vi "Configure QQ.vi"(8 "error in (no error)":errorcluster, 9 "Q / Q High (5 V)":dbl=5.0, 10 "Q / Q Low (0 V)":dbl, 11 "VISA resource name":refnum<visa-resource-name>) -> (0 "error out":errorcluster, 3 "VISA resource name out":refnum<visa-resource-name>)   [LabVIEW 2013, in "Stanford Research CG635.lvlib"]
doc: "Set the Q / Q <b>high</b> and <b>low</b> controls to the specified values.\n\n<b>Note</b>: for standard values/levels, use the Configure Standard Outputs VI."
uses:
  <instrlib>/Stanford Research CG635/Stanford Research CG635.lvlib
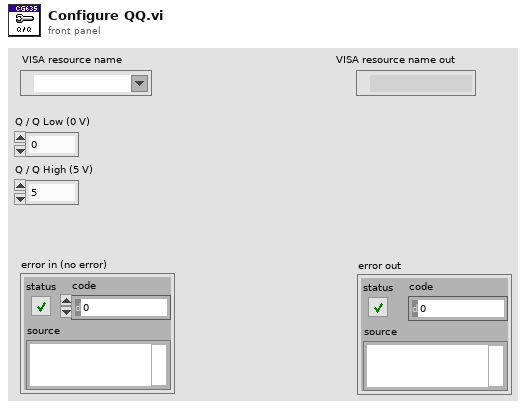
[diagram p1: front panel]
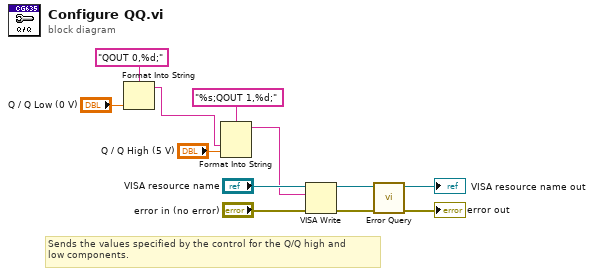
[diagram p0: block diagram]
diagram:
  # "Sends the values specified by the control for the Q/Q high and \nlow components."
  n1 = Format Into String(format string="QOUT 0,%d;", "Q / Q Low (0 V)") -> (resulting string=w6:string)  [unwired: 2 in, 1 out]
  n2 = Format Into String(format string="%s;QOUT 1,%d;", w6, "Q / Q High (5 V)") -> (resulting string=w5:string)  [unwired: 2 in, 1 out]
  n3 = VISA Write(VISA resource name="VISA resource name", write buffer=w5, error in (no error)="error in (no error)") -> (VISA resource name out=w4:refnum<visa-resource-name>, error out=w3:errorcluster)  [unwired: 1 out]
  n4 = call <instrlib>:"Error Query.vi"("error in (no error)"=w3, "VISA resource name"=w4) -> ("error out"=→"error out":errorcluster, "VISA resource name out"=→"VISA resource name out":refnum<visa-resource-name>)  [unwired: 6 in, 2 out]
